vi "RGB LED Configure.vi"(8 "Error In":errorcluster, 10 "RGB LED Pins":T1, 11 "ChipKit Resource":T3={"COM Port"="", "Board Type"=enum."ChipKit uC32", "Connection Type"=enum."USB / Serial", "Baud Rate (115200)"=15, "Bytes Per Packet (15)"=15}) -> (0 "Error Out":errorcluster, 2 "RGB LED Pins":T1, 3 "ChipKit Resource":T3={"COM Port"="", "Board Type"=enum."ChipKit uC32", "Connection Type"=enum."USB / Serial", "Baud Rate (115200)"=15, "Bytes Per Packet (15)"=15})   [LabVIEW 2011, in "LabVIEW Interface for ChipKit.lvlib"]
doc: "Configure Arduino PWM pins for use with an RGB LED."
uses:
  LabVIEW Interface for ChipKit.lvlib
  Private/Type Defs/Chipkit Resource.ctl
  Private/Type Defs/Board Type.ctl
  Private/Type Defs/Connection Type.ctl
  Private/Type Defs/RGB LED Pins.ctl
  Private/Type Defs/PWM Pin.ctl
  Private/Type Defs/Pin Mode.ctl
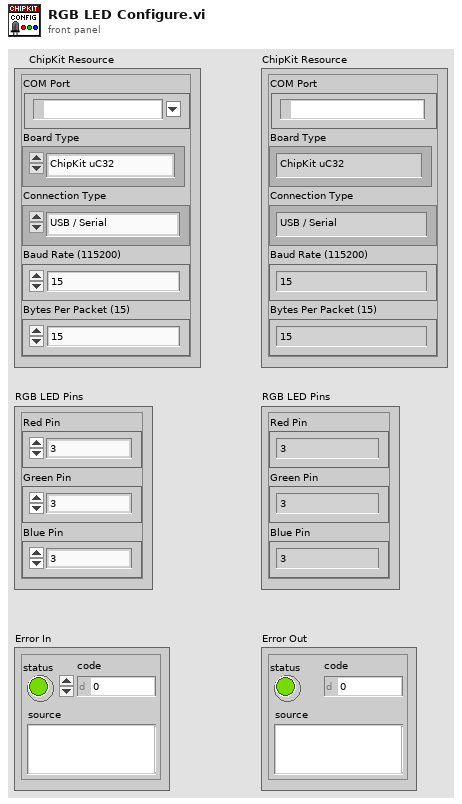
[diagram p1: front panel]
types:
  T1 = typedef "LabVIEW Interface for ChipKit.lvlib/RGB LED Pins.ctl" = cluster{"Red Pin ":T2, "Green Pin":T2, "Blue Pin":T2}
  T2 = typedef "LabVIEW Interface for ChipKit.lvlib/PWM Pin.ctl" = enum8{"3", "5", "6", "9", "10"}
  T3 = typedef "LabVIEW Interface for ChipKit.lvlib/Chipkit Resource.ctl" = cluster{"COM Port":refnum<visa-resource-name>, "Board Type":T4, "Connection Type":T5, "Baud Rate (115200)":u32, "Bytes Per Packet (15)":u32}
  T4 = typedef "LabVIEW Interface for ChipKit.lvlib/Board Type.ctl" = enum16{"ChipKit uC32", "ChipKit Uno32", "ChipKit Max32"}
  T5 = typedef "LabVIEW Interface for ChipKit.lvlib/Connection Type.ctl" = enum8{"USB / Serial", "XBEE", "BlueSmirf (Bluetooth)"}
  T6 = typedef "LabVIEW Interface for ChipKit.lvlib/Pin Mode.ctl" = enum16{"Input", "Output"}
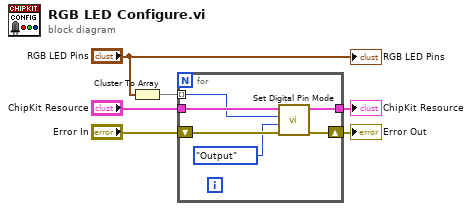
[diagram p0: block diagram]
diagram:
  n1 = Cluster To Array(cluster="RGB LED Pins") -> (array=w1:T2[])
  n2 = for {
    tunnel: "ChipKit Resource" -> [w10]
    shift-right: [w12] -> w5
    shift-left: "Error In" -> [w11]
    tunnel: [w9] -> w3
    tunnel: w1 -> [w7] mode=indexing
    n3 = call "Set Digital Pin Mode.vi"("Error In"=w11, "Pin Mode (Input)"=Pin_Mode."Output", "Digital I/O Pin"=w7, "Arduino Resource"=w10) -> ("Error Out"=w12:errorcluster, "Arduino Resource"=w9:T3)  [unwired: 6 in]
  }
  "Error Out" <- w5
  "ChipKit Resource" <- w3
  "RGB LED Pins" <- "RGB LED Pins"
